vi "Find Galaxies.vi"(11 "Universe In":string[][](array[string])) -> (3 "Galaxies":cluster{"x":i32, "y":i32}[](array[cluster]))   [LabVIEW 2021]
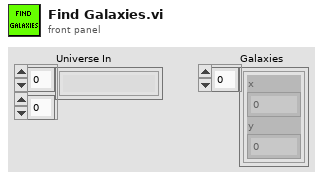
[diagram p1: front panel]
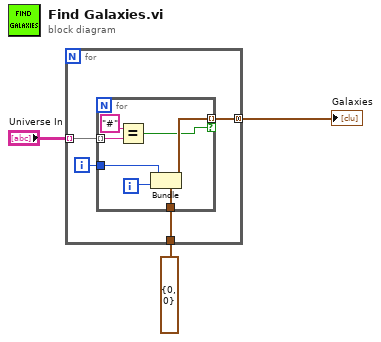
[diagram p0: block diagram]
diagram:
  n1 = for {
    tunnel: "Universe In" -> [w7] mode=indexing
    tunnel: [w5] -> w3 mode=concatenating
    tunnel: cluster{"x":i32, "y":i32} {"x"=0, "y"=0} ("cluster") -> [w4]
    i -> [w6]
    n2 = for {
      tunnel: w7 -> [w14] mode=indexing
      tunnel: w6 -> [w11]
      tunnel: [w10] -> w5 mode=indexing if=w9
      tunnel: w4 -> [w8]
      i -> [w12]
      n3 = Equal?(x="#", y=w14) -> (x = y?=w9:bool)
      n4 = Bundle(cluster=w8, "x"=w11, "y"=w12) -> (w10:cluster{"x":i32, "y":i32})
    }
  }
  "Galaxies" <- w3
